vi "STAGE+mono+counter.vi"() -> ()   [LabVIEW 2017]
panel:
  out "Current WL Wavelength  2":u16 caption="Current Wavelength"
  out "Grt# 2":u8=1 min=1 max=3 step=1
  out "Blaze (nm) 2":u32=300
  out "Groove/mm 2":u32=1200
  in  "?":bool
  in  "Channel B Input":u16(ring)=2 items=["Input 1"=1, "Input 2"=2]
  in  "Trigger mode":u16(ring) items=["10 MHz"=0, "Input 2"=2, "Input T"=3]
  out "Current WL Wavelength":u16 caption="Current Wavelength"
  in  "Integrating time, 10^-7 sec":dbl=10000000.0
  in  "gate A mode (CW:0)":i16(slide) scale=0.0..2.0 scale format="%.2f"
  in  "Channel A Input":u16(ring)=1 items=["10 MHz", "Input 1"]
  in  "Time between measurements\n at one point (s)/Dwell Time":dbl=0.002 min=0.002 max=60.0 step=0.001
  in  "Number of Measurements\n to take at one point/ Number of Periods":u16=1 min=1 max=2000 step=1
  in  "Count Mode":u16(ring) items=["A,B for Preset T", "A-B for Preset T", "A+B for Preset T", "A for Preset B"]
  in  "GPIB address":string="23"
  out "Timeout":bool
  out "Serial":u32=12345
  out "Grt#":u8=1 min=1 max=3 step=1
  out "Blaze (nm)":u32=300
  out "Groove/mm":u32=1200
  out "time delay":u32=450000 min=1
  out "Mono port":T1(ring)
  in  "Get position":bool
  out "Position status":dbl format="%.3f"
  in  "Target position":dbl format="%.3f"
  in  "Move":bool
  in  "Motor OFF":bool
  in  "Motor ON":bool
  in  "Step Size [um]":i32=10
  in  "Axis":i32=1
  in  "Rep Rate [Hz]":dbl=500.0
  out "Shots":dbl
  in  "Averaging Time [s]":dbl=0.1
  out "Current Point":i32
  out "Slide":i32(slide) scale=0.0..100.0
  out "Current Position [mm]":dbl
  in  "Axis initial position [mm]":dbl
  out "Axis final Position [mm]":dbl
  in  "Data Points (100 default)":i32=100
  in  "Collect Data!":bool
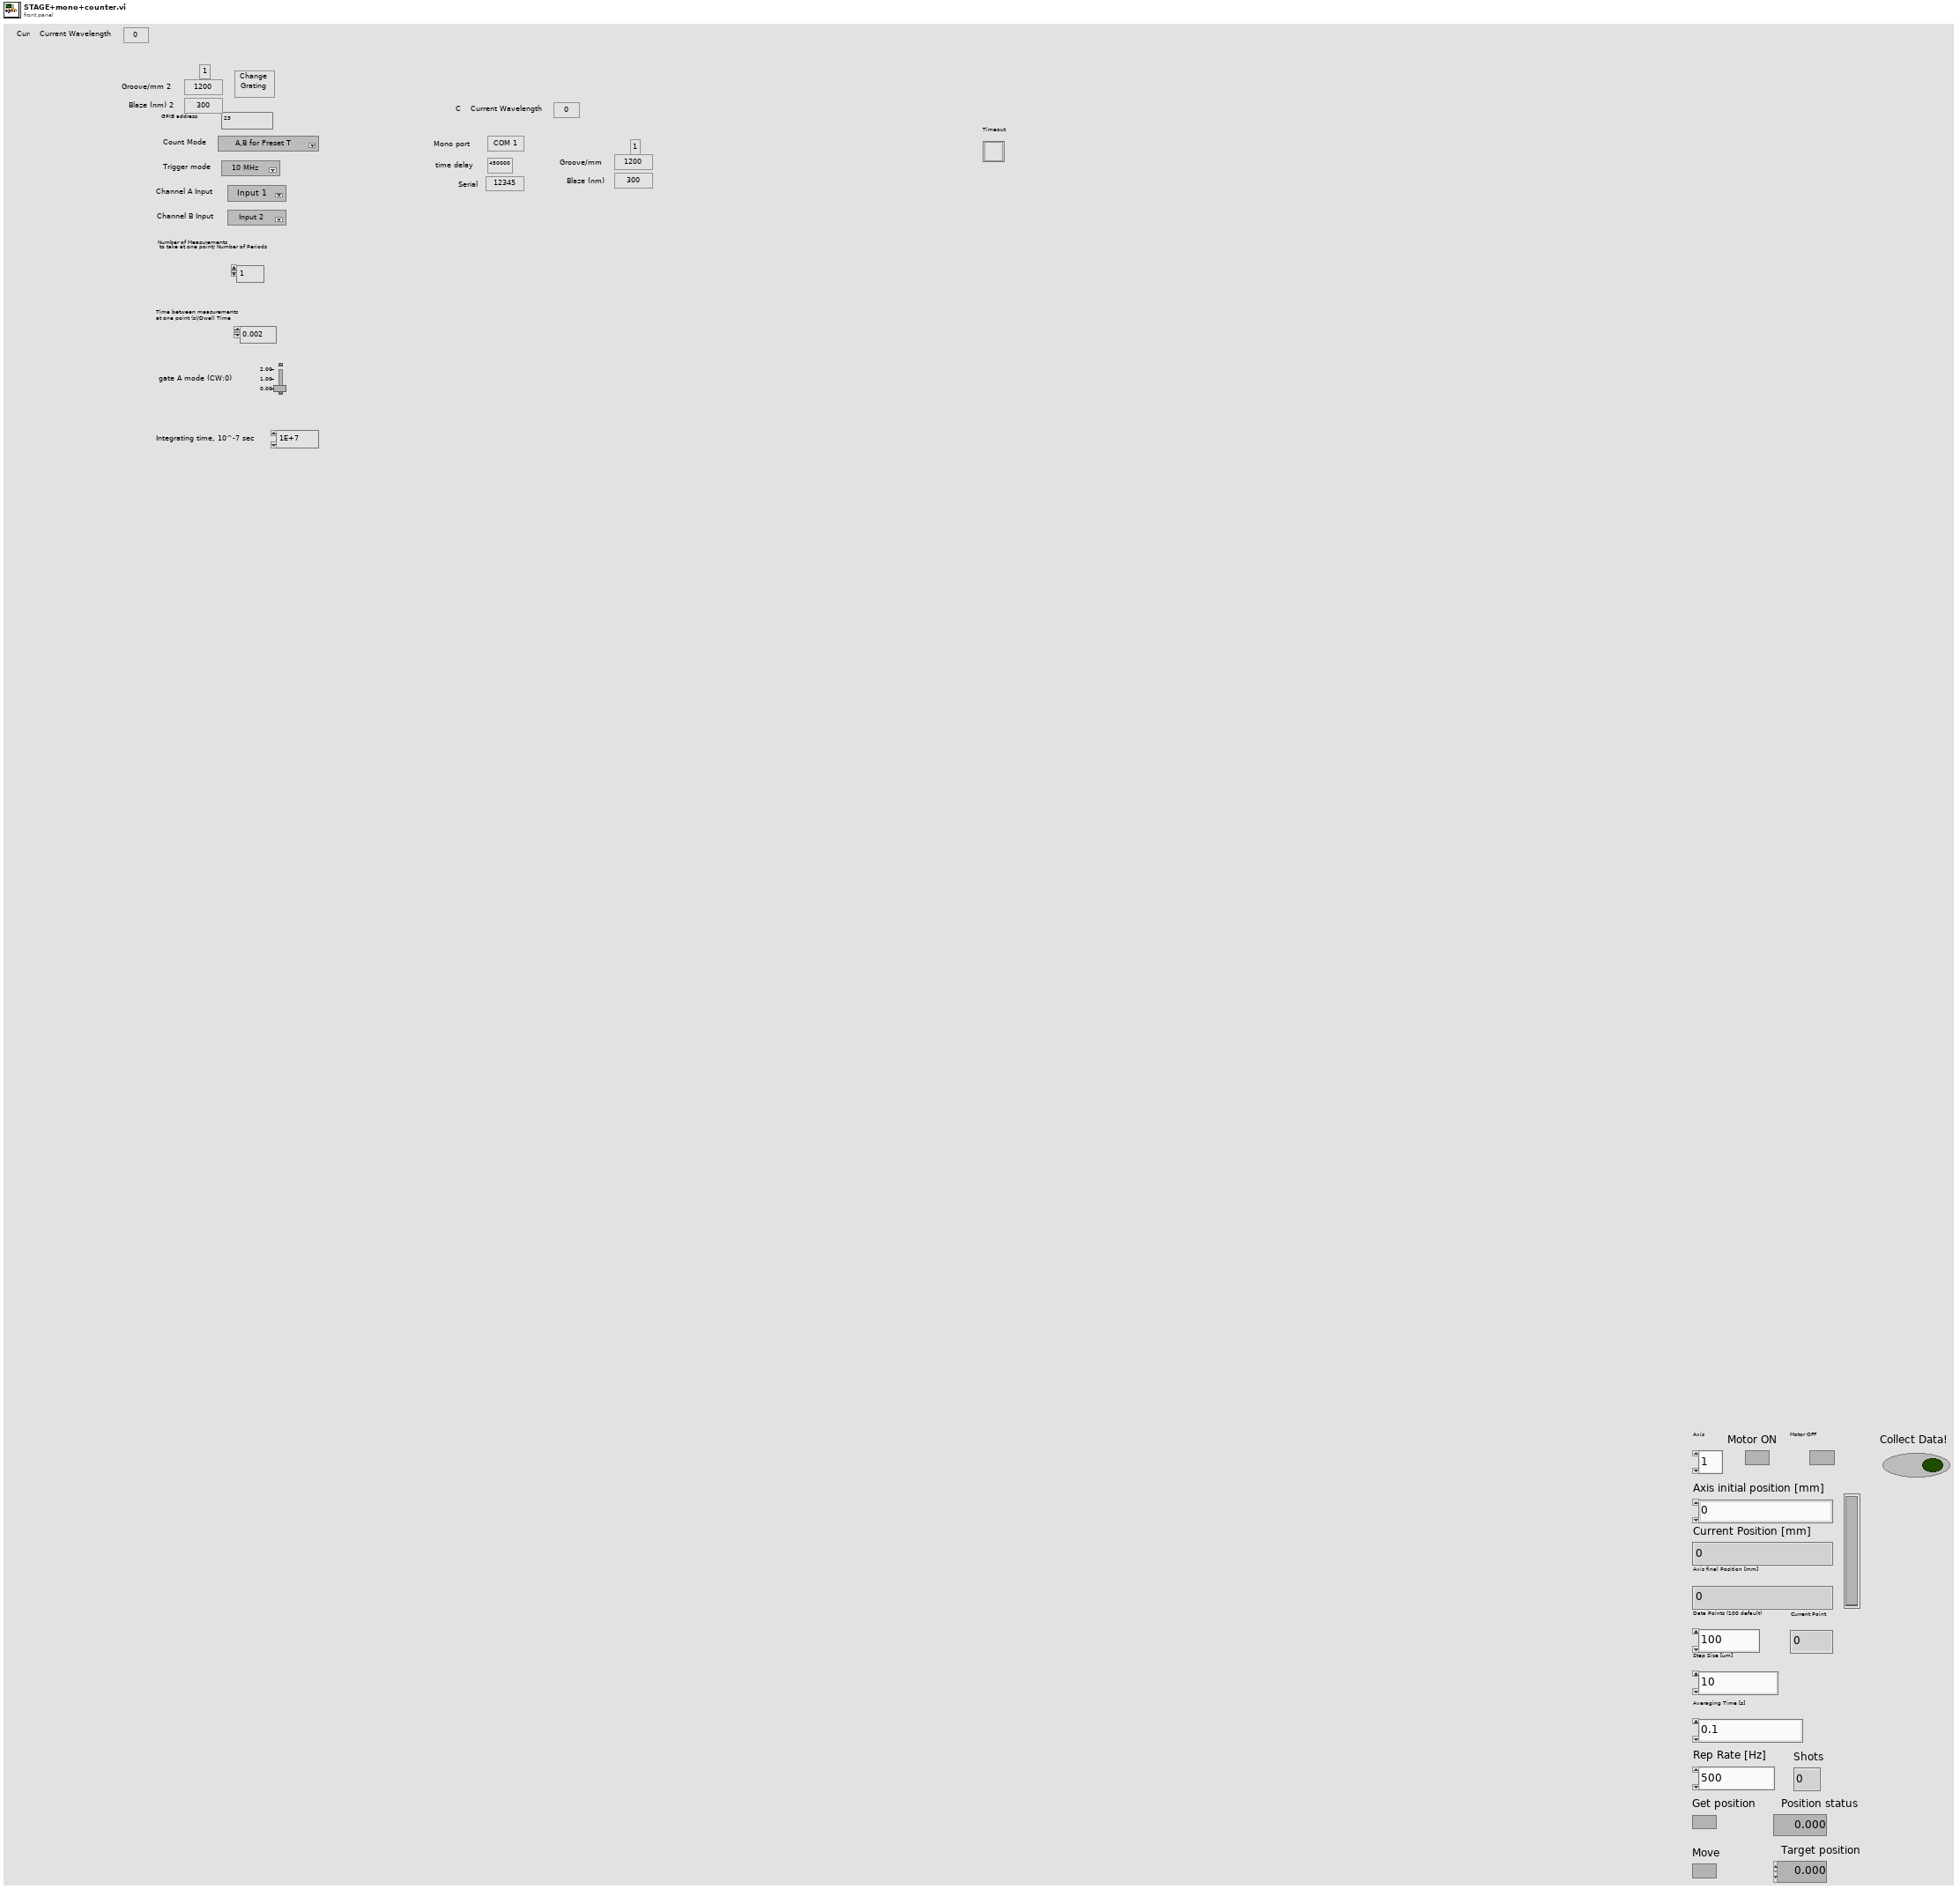
[diagram p1: front panel]
types:
  T1 = enum8{"COM 1", "COM 2", "COM 3", "COM 4", "COM 5", "COM 6", "COM 7", "COM 8", "COM 9"}
  T2 = cluster{"input XON/XOFF":bool, "input HW Handshake":bool, "input alt HW HShk":bool, "output XON/XOFF":bool, "output HW Handshake":bool, "output alt HW HShk":bool, "XOFF byte":u8, "XON byte":u8, "parity error byte":u16}
  T3 = enum16{"no parity", "odd parity", "even parity", "mark parity", "space parity"}
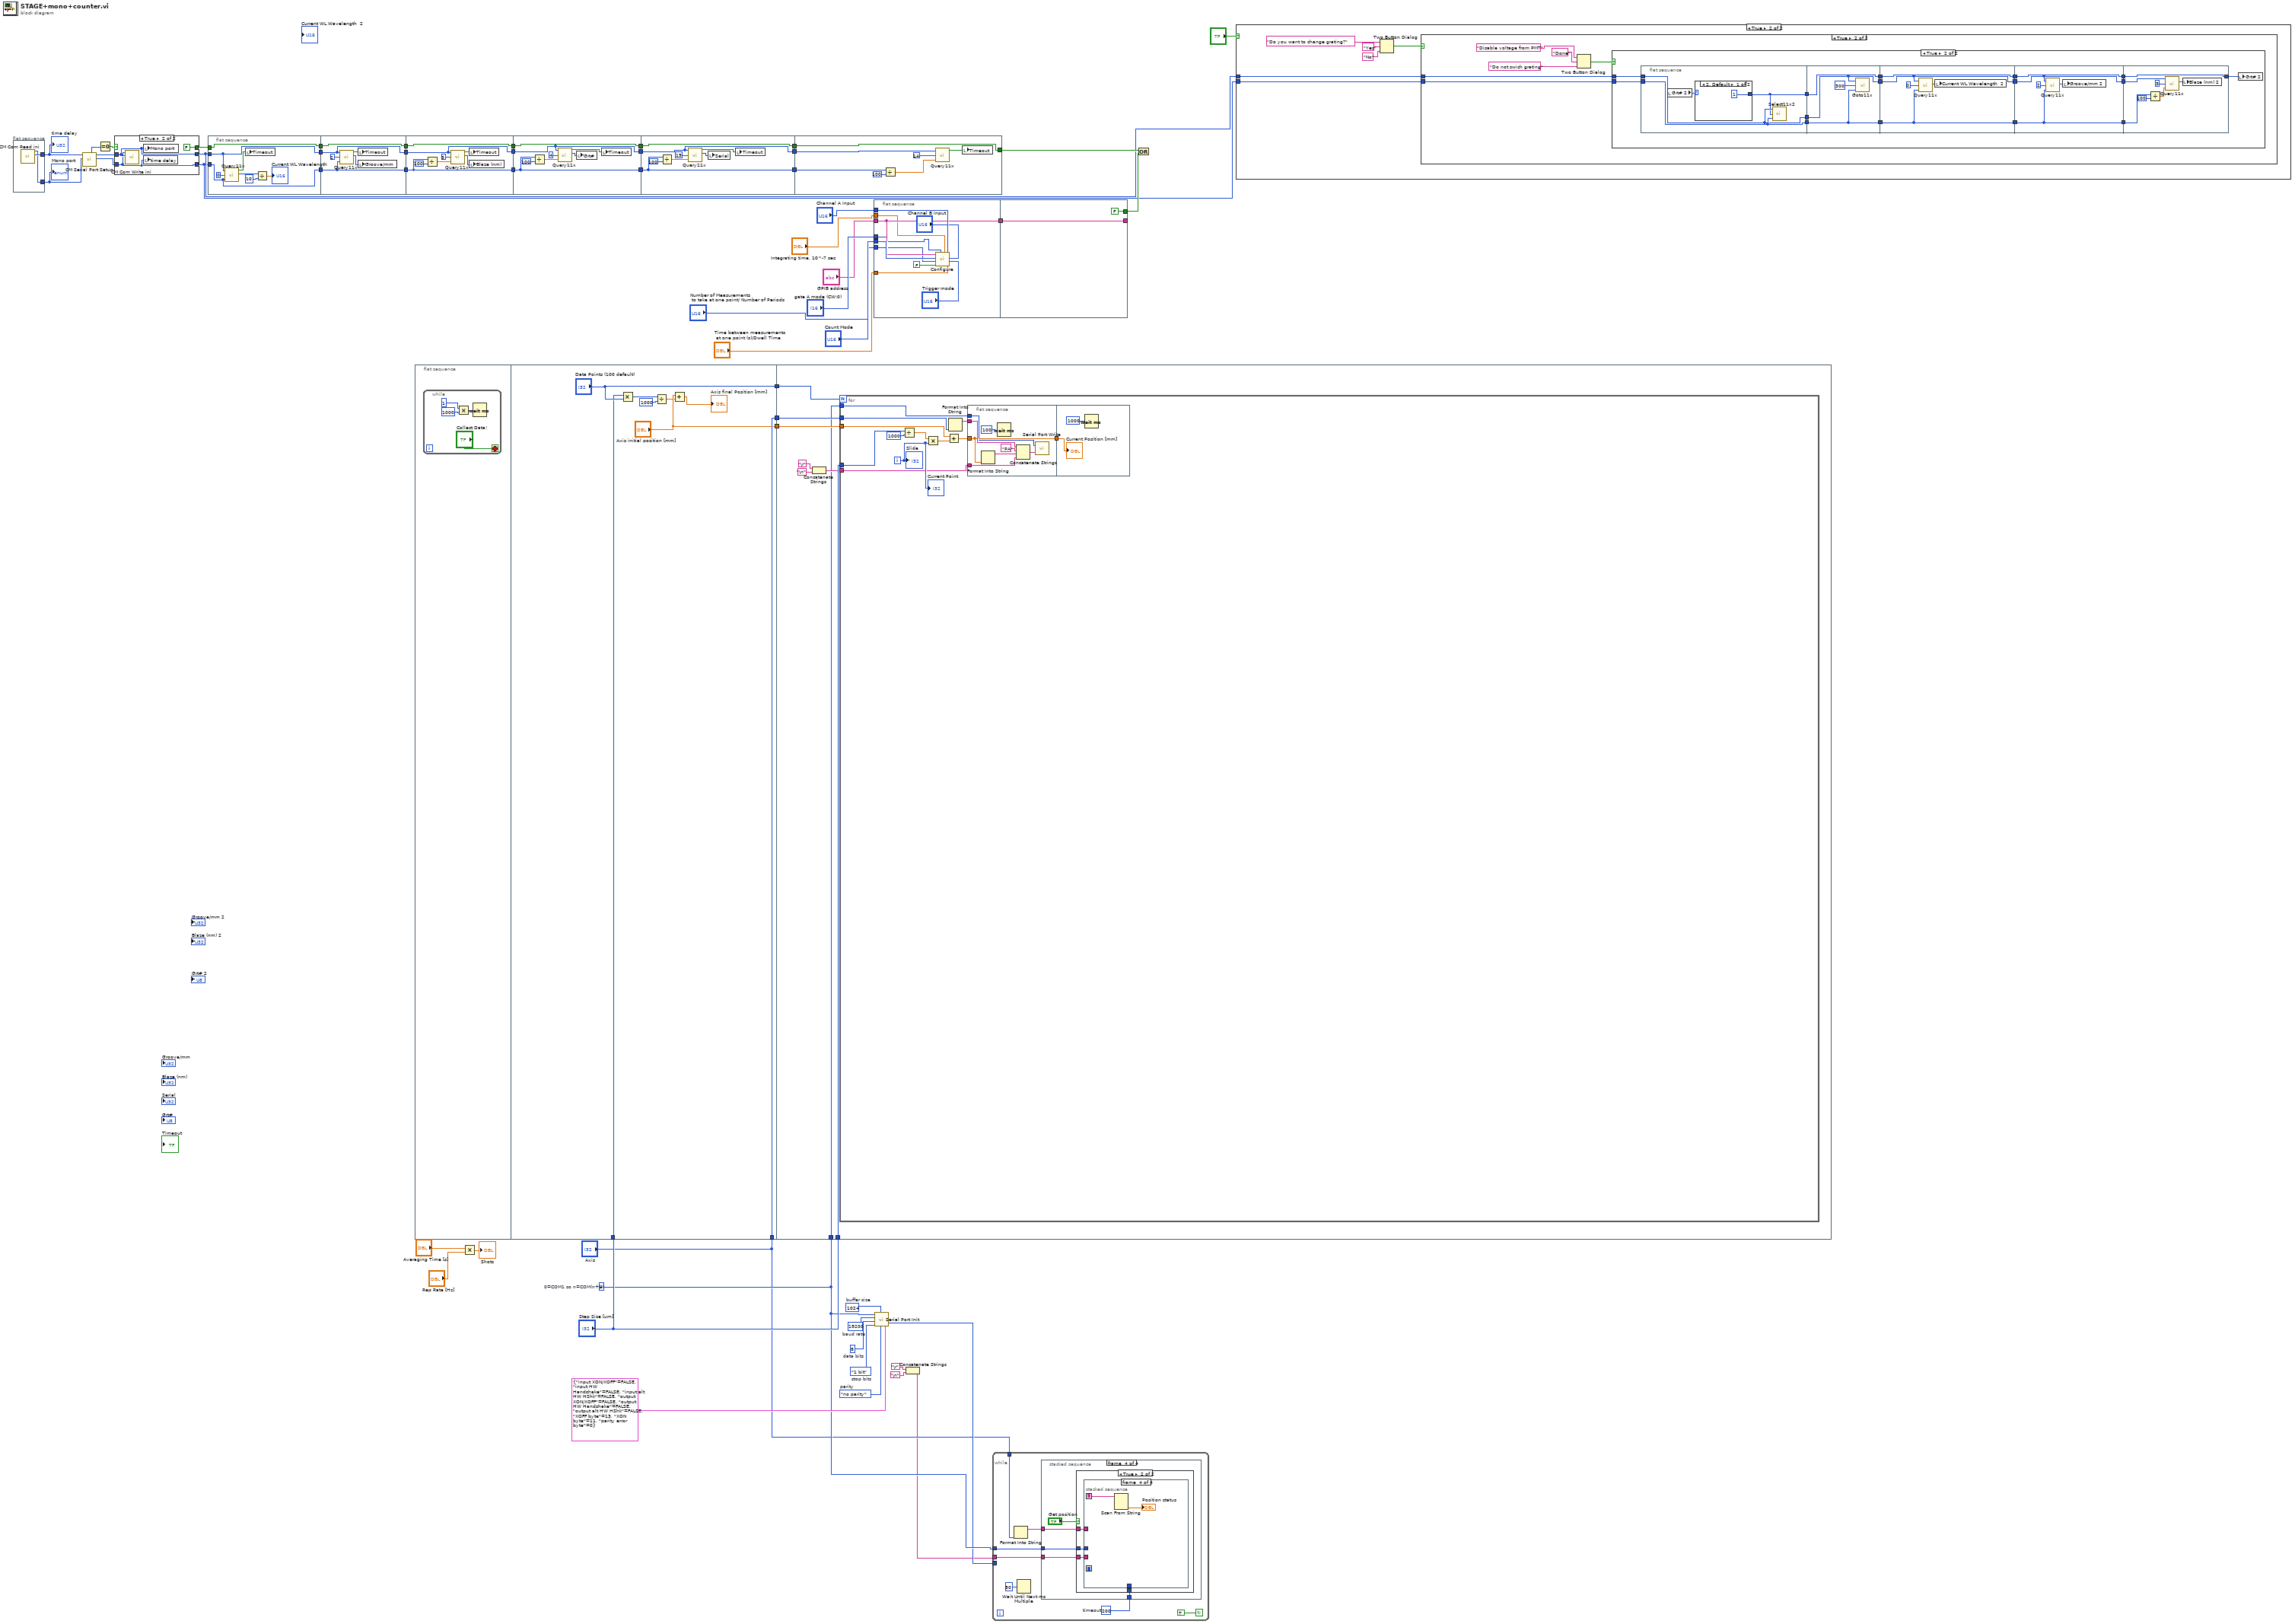
[diagram p0: block diagram]
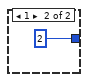
[diagram p5: hidden frame]
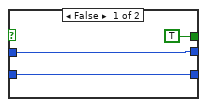
[diagram p6: hidden frame]
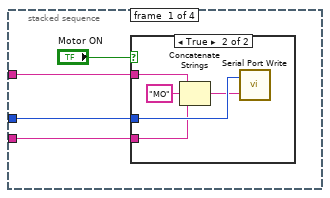
[diagram p7: hidden frame]
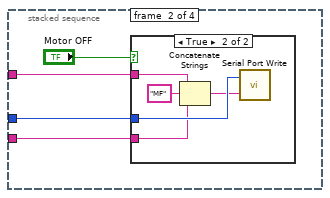
[diagram p9: hidden frame]
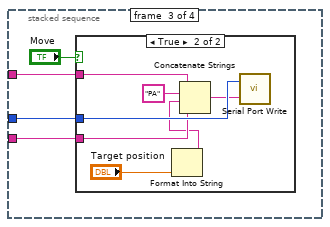
[diagram p11: hidden frame]
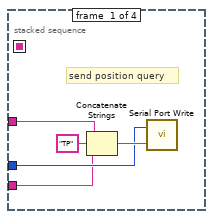
[diagram p14: hidden frame]
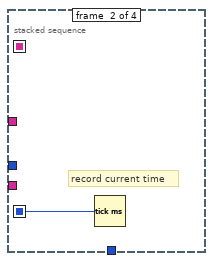
[diagram p15: hidden frame]
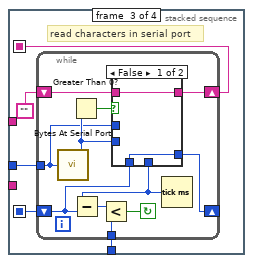
[diagram p16: hidden frame]
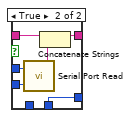
[diagram p17: hidden frame]
diagram:
  w44 = u32 19200  # baud rate
  w43 = u16 8  # data bits
  w42 = enum16{"1 bit", "1.5 bits", "2 bits"}."1 bit"  # stop bits
  w47 = T3."no parity"  # parity
  w41 = 4  # 0=COM1 so n=COM(n+1)
  w46 = u16 1024  # buffer size
  n1 = flat-sequence {
    tunnel: [w56] -> w19
    tunnel: [w55] -> w18
    frame #0 {
      n2 = call "CM Com Read ini.vi"() -> ("Mono port"=w55:T1, "time delay1"=w56:u32)  [unwired: 7 in]
    }
  }
  n3 = call "CM Serial Port Setup.vi"("COM port"=w18, "time delay"=w19) -> ("time delay1"=w14:u32, "DK port Out"=w15:T1, "error code"=w17:i32)  [unwired: 7 in]
  n4 = Equal To 0?(x=w17) -> (x = 0?=w16:bool)
  n5 = case shown="True" w16 {
    tunnel: w15 -> [w59 w62]
    tunnel: w14 -> [w58 w61]
    tunnel: [w59 w62] -> w2
    tunnel: [w58 w61] -> w1
    tunnel: [TRUE FALSE] -> w13
    frame False {
    }
    frame True {
      n6 = call "CM Com Write ini.vi"("time delay1"=w62, "Mono port"=w61) -> ()  [unwired: 7 in]
      n7 = local write "Mono port"(w62) -> ()
      n8 = local write "time delay"(w61) -> ()
    }
  }
  n9 = flat-sequence {
    tunnel: w1 -> [w68]
    tunnel: [w68] -> w35
    tunnel: w2 -> [w70]
    tunnel: [w70] -> w34
    tunnel: w13 -> [w66]
    tunnel: [w66] -> w33
    tunnel: w35 -> [w73]
    tunnel: [w73] -> w32
    tunnel: w34 -> [w75]
    tunnel: [w75] -> w31
    tunnel: w33 -> [w71]
    tunnel: [w71] -> w30
    tunnel: w32 -> [w83]
    tunnel: [w83] -> w29
    tunnel: w31 -> [w80]
    tunnel: [w80] -> w28
    tunnel: w30 -> [w77]
    tunnel: [w77] -> w27
    tunnel: w29 -> [w91]
    tunnel: [w91] -> w26
    tunnel: w28 -> [w88]
    tunnel: [w88] -> w25
    tunnel: w27 -> [w85]
    tunnel: [w85] -> w24
    tunnel: w26 -> [w99]
    tunnel: [w99] -> w23
    tunnel: w25 -> [w96]
    tunnel: [w96] -> w22
    tunnel: w24 -> [w93]
    tunnel: [w93] -> w21
    tunnel: w23 -> [w106]
    tunnel: w22 -> [w103]
    tunnel: [w101] -> w7
    tunnel: w21 -> [w101]
    frame #0 {
      n10 = call "Query11x.vi"("port number"=w70, "QUERY"=u16 0, "time delay"=w68) -> ("timeout"=w67:bool, "STATUS MESSAGE"=w65:u16)  [unwired: 2 out]
      n11 = local write "Timeout"(w67) -> ()
      n12 = Divide(x=w65, y=10 ("Numeric")) -> (x/y=→"Current WL Wavelength":dbl)
    }
    frame #1 {
      n13 = call "Query11x.vi"("port number"=w75, "QUERY"=u16 2, "time delay"=w73) -> ("timeout"=w72:bool, "STATUS MESSAGE"=w74:u16)  [unwired: 2 out]
      n14 = local write "Timeout"(w72) -> ()
      n15 = local write "Groove/mm"(w74) -> ()
    }
    frame #2 {
      n16 = Divide(x=w83, y=i16 100 ("device (1)")) -> (x/y=w81:dbl)
      n17 = call "Query11x.vi"("port number"=w80, "QUERY"=u16 3, "time delay"=w81) -> ("timeout"=w78:bool, "STATUS MESSAGE"=w79:u16)  [unwired: 2 out]
      n18 = local write "Timeout"(w78) -> ()
      n19 = local write "Blaze (nm)"(w79) -> ()
    }
    frame #3 {
      n20 = Divide(x=w91, y=i16 100 ("device (1)")) -> (x/y=w89:dbl)
      n21 = call "Query11x.vi"("port number"=w88, "QUERY"=u16 4, "time delay"=w89) -> ("timeout"=w86:bool, "STATUS MESSAGE"=w87:u16)  [unwired: 2 out]
      n22 = local write "Grt#"(w87) -> ()
      n23 = local write "Timeout"(w86) -> ()
    }
    frame #4 {
      n24 = Divide(x=w99, y=i16 100 ("device (1)")) -> (x/y=w97:dbl)
      n25 = call "Query11x.vi"("port number"=w96, "QUERY"=u16 19, "time delay"=w97) -> ("timeout"=w94:bool, "STATUS MESSAGE"=w95:u16)  [unwired: 2 out]
      n26 = local write "Serial"(w95) -> ()
      n27 = local write "Timeout"(w94) -> ()
    }
    frame #5 {
      n28 = Divide(x=w106, y=i16 100 ("device (1)")) -> (x/y=w104:dbl)
      n29 = call "Query11x.vi"("port number"=w103, "QUERY"=u16 14, "time delay"=w104) -> ("timeout"=w102:bool)  [unwired: 3 out]
      n30 = local write "Timeout"(w102) -> ()
    }
  }
  n31 = flat-sequence {
    tunnel: ["Data Points (100 default)"] -> w54
    tunnel: "Axis" -> [w119]
    tunnel: ["Axis initial position [mm]"] -> w53
    tunnel: "Step Size [um]" -> [w112]
    tunnel: [w119] -> w52
    tunnel: w54 -> [w127]
    tunnel: w53 -> [w126]
    tunnel: "Step Size [um]" -> [w125]
    tunnel: w52 -> [w124]
    tunnel: w41 -> [w120]
    frame #0 {
      n32 = while {
        stop <- "Collect Data!" stop-if-true
        n33 = Multiply(x=1, y=1000) -> (x*y=w111:i32)
        n34 = Wait (ms)(milliseconds to wait=w111) -> ()  [unwired: 1 out]
      }
    }
    frame #1 {
      n35 = Multiply(x=w112, y="Data Points (100 default)") -> (x*y=w115:i32)
      n36 = Divide(x=w115, y=1000) -> (x/y=w114:dbl)
      n37 = Add(x="Axis initial position [mm]", y=w114) -> (x+y=→"Axis final Position [mm]":dbl)
    }
    frame #2 {
      n38 = Concatenate Strings("\r", "\n") -> (w121:string)
      n39 = for {
        N: w127 -> [_]
        tunnel: w126 -> [w138]
        tunnel: w125 -> [w134]
        tunnel: w124 -> [w131]
        tunnel: w121 -> [w128]
        tunnel: w120 -> [w129]
        i -> [w139]
        n40 = Divide(x=w134, y=1000) -> (x/y=w133:dbl)
        n41 = Multiply(x=w133, y=w139) -> (x*y=w137:dbl)
        n42 = Add(x=w138, y=w137) -> (x+y=w136:dbl)
        n43 = Format Into String(w131) -> (resulting string=w130:string)  [unwired: 3 in, 1 out]
        n44 = flat-sequence {
          tunnel: w136 -> [w142]
          tunnel: [w142] -> w132
          tunnel: w128 -> [w144]
          tunnel: w130 -> [w143]
          tunnel: w129 -> [w140]
          tunnel: w132 -> [w148]
          frame #0 {
            n45 = Format Into String(w142) -> (resulting string=w141:string)  [unwired: 3 in, 1 out]
            n46 = Wait (ms)(milliseconds to wait=u32 100) -> ()  [unwired: 1 out]
            n47 = Concatenate Strings(w143, "PA" ("Substring"), w141, w144) -> (w146:string)
            n48 = call <vilib>:"Serial Port Write.vi"("string to write"=w146, "port number"=w140) -> ()  [unwired: 1 out]
          }
          frame #1 {
            n49 = Wait (ms)(milliseconds to wait=u32 1000) -> ()  [unwired: 1 out]
            "Current Position [mm]" <- w148
          }
        }
        "Current Point" <- w139
        "Slide" <- w139
      }
    }
  }
  n50 = Multiply(x="Averaging Time [s]", y="Rep Rate [Hz]") -> (x*y=→"Shots":dbl)
  n51 = flat-sequence {
    tunnel: "GPIB address" -> [w157]
    tunnel: [w157] -> w20
    tunnel: "Count Mode" -> [w158]
    tunnel: "Number of Measurements\n to take at one point/ Number of Periods" -> [w155]
    tunnel: "Time between measurements\n at one point (s)/Dwell Time" -> [w154]
    tunnel: "Channel A Input" -> [w159]
    tunnel: "gate A mode (CW:0)" -> [w151]
    tunnel: "Integrating time, 10^-7 sec" -> [w150]
    tunnel: w20 -> [w160]
    tunnel: [w160] -> _
    tunnel: [FALSE] -> w8
    frame #0 {
      n52 = call "Configure.vi"("Dwell Time (s)"=w154, "Channel T Input"="Trigger mode", "Channel B Input"="Channel B Input", "Channel A Input"=w159, "Integrating time, 10^-7 sec"=w150, "gate mode (CW:0)"=w151, "Scan End Mode"=FALSE, "Number of Periods"=w155, "Count Mode"=w158, "GPIB Address"=w157) -> ()
    }
    frame #1 {
    }
  }
  n53 = call <vilib>:"Serial Port Init.vi"("flow control etc."=T2 {"input XON/XOFF"=FALSE, "input HW Handshake"=FALSE, "input alt HW HShk"=FALSE, "output XON/XOFF"=FALSE, "output HW Handshake"=FALSE, "output alt HW HShk"=FALSE, "XOFF byte"=13, "XON byte"=11, "parity error byte"=0}, "parity"=w47, "buffer size"=w46, "stop bits"=w42, "data bits"=w43, "baud rate"=w44, "port number"=w41) -> ("error code"=w40:i32)
  n54 = Concatenate Strings("\r", "\n") -> (w36:string)
  n55 = while {
    tunnel: w41 -> [w164]
    tunnel: w36 -> [w165]
    tunnel: w40 -> [_]
    tunnel: "Axis" -> [w162]
    stop <- TRUE continue-if-true
    w163 = u32 200  # timeout
    n56 = Format Into String(w162) -> (resulting string=w166:string)  [unwired: 3 in, 1 out]
    n57 = Wait Until Next ms Multiple(millisecond multiple=u32 50) -> ()  [unwired: 1 out]
    n58 = stacked-sequence {
      tunnel: w166 -> [w170 w180 w189 w201]
      tunnel: w165 -> [w169 w179 w188 w198]
      tunnel: w164 -> [w171 w181 w190 w200]
      tunnel: w163 -> [_ _ _ w199]
      frame #0 {
        n59 = case shown="True" "Motor ON" {
          tunnel: w171 -> [_ w177]
          tunnel: w170 -> [_ w174]
          tunnel: w169 -> [_ w173]
          frame False {
          }
          frame True {
            n60 = Concatenate Strings(w174, "MO" ("Substring"), w173) -> (w175:string)
            n61 = call <vilib>:"Serial Port Write.vi"("string to write"=w175, "port number"=w177) -> ()  [unwired: 1 out]
          }
        }
      }
      frame #1 {
        n62 = case shown="True" "Motor OFF" {
          tunnel: w181 -> [_ w186]
          tunnel: w180 -> [_ w183]
          tunnel: w179 -> [_ w182]
          frame False {
          }
          frame True {
            n63 = Concatenate Strings(w183, "MF" ("Substring"), w182) -> (w184:string)
            n64 = call <vilib>:"Serial Port Write.vi"("string to write"=w184, "port number"=w186) -> ()  [unwired: 1 out]
          }
        }
      }
      frame #2 {
        n65 = case shown="True" "Move" {
          tunnel: w190 -> [_ w197]
          tunnel: w189 -> [_ w194]
          tunnel: w188 -> [_ w193]
          frame False {
          }
          frame True {
            n66 = Format Into String("Target position") -> (resulting string=w191:string)  [unwired: 3 in, 1 out]
            n67 = Concatenate Strings(w194, "PA" ("Substring"), w191, w193) -> (w195:string)
            n68 = call <vilib>:"Serial Port Write.vi"("string to write"=w195, "port number"=w197) -> ()  [unwired: 1 out]
          }
        }
      }
      frame #3 {
        n69 = case shown="True" "Get position" {
          tunnel: w201 -> [_ w206]
          tunnel: w200 -> [_ w205]
          tunnel: w199 -> [_ w204]
          tunnel: w198 -> [_ w203]
          frame False {
          }
          frame True {
            n70 = stacked-sequence {
              seq-local: [_ w212 _ _] -> [_ _ w214 _]
              seq-local: [_ _ w213 _] -> [_ _ _ w238]
              tunnel: w206 -> [w209 _ _ _]
              tunnel: w205 -> [w208 _ w217 _]
              tunnel: w204 -> [_ _ w215 _]
              tunnel: w203 -> [w207 _ _ _]
              frame #0 {
                # "send position query"
                n71 = Concatenate Strings(w209, "TP" ("Substring"), w207) -> (w210:string)
                n72 = call <vilib>:"Serial Port Write.vi"("string to write"=w210, "port number"=w208) -> ()  [unwired: 1 out]
              }
              frame #1 {
                # "record current time"
                n73 = Tick Count (ms)() -> (millisecond timer value=w212:u32)
              }
              frame #2 {
                # "read characters in serial port"
                n74 = while {
                  shift-left: w214 -> [w218]
                  shift-right: [w219] -> _
                  tunnel: w215 -> [w222]
                  shift-left: "" -> [w225]
                  shift-right: [w224] -> w213
                  tunnel: w217 -> [w226]
                  stop <- w221 continue-if-true
                  n75 = call <vilib>:"Bytes At Serial Port.vi"("port number"=w226) -> ("byte count"=w227:u32)  [unwired: 1 out]
                  n76 = Greater Than 0?(x=w227) -> (x > 0?=w228:bool)
                  n77 = Tick Count (ms)() -> (millisecond timer value=w220:u32)
                  n78 = Subtract(x=w220, y=w218) -> (x-y=w223:u32)
                  n79 = Less?(x=w223, y=w222) -> (x < y?=w221:bool)
                  n80 = case shown="False" w228 {
                    tunnel: w227 -> [_ w236]
                    tunnel: w226 -> [_ w235]
                    tunnel: w225 -> [w230 w233]
                    tunnel: [w230 w232] -> w224
                    tunnel: [w229 w231] -> w219
                    tunnel: w220 -> [_ w231]
                    tunnel: w218 -> [w229 _]
                    frame False {
                    }
                    frame True {
                      n81 = call <vilib>:"Serial Port Read.vi"("requested byte count"=w236, "port number"=w235) -> ("string read"=w234:string)  [unwired: 1 out]
                      n82 = Concatenate Strings(w233, w234) -> (w232:string)
                    }
                  }
                }
              }
              frame #3 {
                n83 = Scan From String(input string=w238) -> (output 1=→"Position status":dbl)  [unwired: 4 in, 3 out]
              }
            }
          }
        }
      }
    }
  }
  n84 = Or(x=w7, y=w8) -> ()  [unwired: 1 out]
  n85 = case shown="True" "?" {
    tunnel: w1 -> [_ w240]
    tunnel: w2 -> [_ w239]
    frame False {
    }
    frame True {
      n86 = Two Button Dialog(message="Do you want to change grating?", 1:"No" ("F button name (\"Cancel\")"), 2:"Yes" ("T button name (\"OK\")")) -> (T button?=w241:bool)
      n87 = case shown="True" w241 {
        tunnel: w240 -> [_ w246]
        tunnel: w239 -> [_ w245]
        frame False {
        }
        frame True {
          n88 = Two Button Dialog(message="Disable voltage from PMT", 1:"Do not swich grating" ("F button name (\"Cancel\")"), 2:"Done" ("T button name (\"OK\")")) -> (T button?=w247:bool)
          n89 = case shown="True" w247 {
            tunnel: w246 -> [_ w265]
            tunnel: w245 -> [_ w264]
            frame False {
            }
            frame True {
              n90 = flat-sequence {
                tunnel: w265 -> [w269]
                tunnel: [w269] -> w262
                tunnel: w264 -> [w268]
                tunnel: [w268] -> w261
                tunnel: [w266] -> w260
                tunnel: w262 -> [w273]
                tunnel: [w273] -> w259
                tunnel: w261 -> [w274]
                tunnel: [w274] -> w258
                tunnel: w260 -> [w272]
                tunnel: [w272] -> w257
                tunnel: w259 -> [w280]
                tunnel: [w280] -> w256
                tunnel: w258 -> [w279]
                tunnel: [w279] -> w255
                tunnel: w257 -> [w276]
                tunnel: [w276] -> w254
                tunnel: w256 -> [w283]
                tunnel: [w283] -> w253
                tunnel: w255 -> [w284]
                tunnel: [w284] -> w252
                tunnel: w254 -> [w281]
                tunnel: [w281] -> w251
                tunnel: w253 -> [w288]
                tunnel: w252 -> [w289]
                tunnel: [w286] -> w263
                tunnel: w251 -> [w286]
                frame #0 {
                  n91 = local read "Grt# 2"() -> (w267:u8)
                  n92 = case shown="2, Default" w267 {
                    tunnel: [1 2] -> w266
                    frame 2, Default {
                    }
                    frame 1 {
                    }
                  }
                  n93 = call "Select11x2.vi"("time delay"=w269, "NEW GRT?"=w266, "port number"=w268) -> ()  [unwired: 3 out]
                }
                frame #1 {
                  n94 = call "Goto11x.vi"("time delay"=w273, "WAVELENGTH"=u16 300, "port number"=w274) -> ()  [unwired: 3 out]
                }
                frame #2 {
                  n95 = call "Query11x.vi"("port number"=w279, "QUERY"=u16 0, "time delay"=w280) -> ("STATUS MESSAGE"=w277:u16)  [unwired: 3 out]
                  n96 = local write "Current WL Wavelength  2"(w277) -> ()
                }
                frame #3 {
                  n97 = call "Query11x.vi"("port number"=w284, "QUERY"=u16 2, "time delay"=w283) -> ("STATUS MESSAGE"=w282:u16)  [unwired: 3 out]
                  n98 = local write "Groove/mm 2"(w282) -> ()
                }
                frame #4 {
                  n99 = Divide(x=w288, y=i16 100 ("device (1)")) -> (x/y=w290:dbl)
                  n100 = call "Query11x.vi"("port number"=w289, "QUERY"=u16 3, "time delay"=w290) -> ("STATUS MESSAGE"=w287:u16)  [unwired: 3 out]
                  n101 = local write "Blaze (nm) 2"(w287) -> ()
                }
              }
              n102 = local write "Grt# 2"(w263) -> ()
            }
          }
        }
      }
    }
  }
  "Mono port" <- w18
  "time delay" <- w19
